vi "Configure Current Limit.vi"(8 "error in (no error)":errorcluster, 10 "Current Limit":dbl, 11 "Agilent 6xxx in":refnum<class "Agilent 6xxx.lvclass">) -> (0 "error out":errorcluster, 3 "Agilent 6xxx out":refnum<class "Agilent 6xxx.lvclass">)   [LabVIEW 2020, in "Agilent 6xxx.lvclass"]
uses:
  Agilent 6xxx.lvclass
  C:/Sandbox/RF Bench/Source Code/WiSpry Test Framework/Instruments/Instrument.lvclass
  C:/Sandbox/RF Bench/Source Code/WiSpry Test Framework/Instruments/Power Supply/Power Supply.lvclass
  Power Supply.lvclass/Power Supply.ctl
  Instrument.lvclass/Instrument.ctl
  Power Supply.lvclass
  Instrument.lvclass
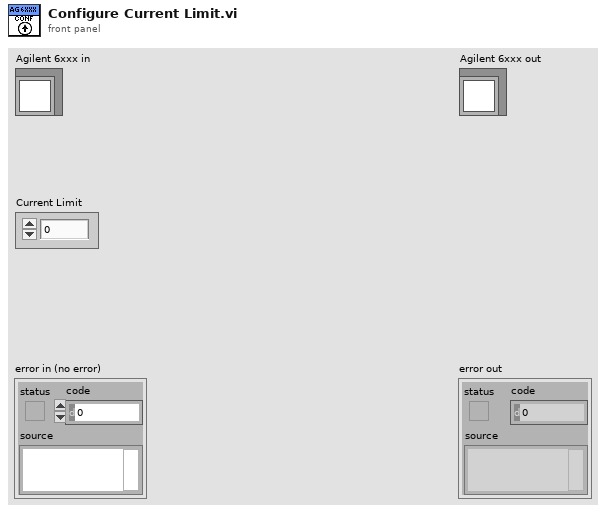
[diagram p1: front panel]
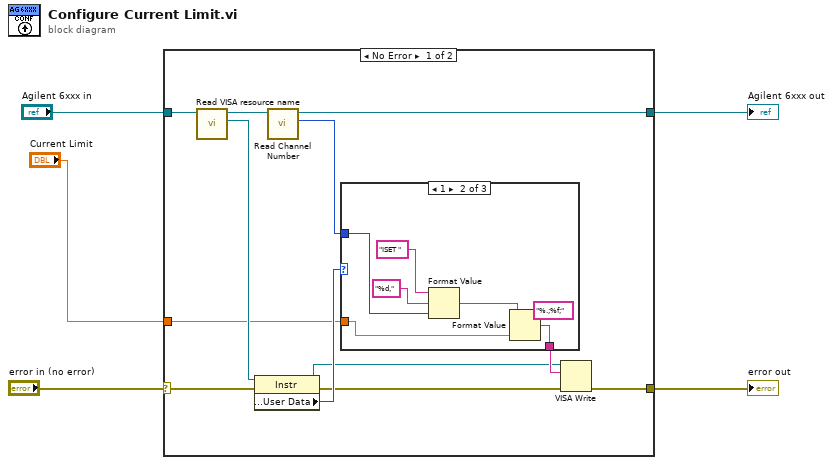
[diagram p0: block diagram]
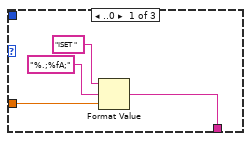
[diagram p2: hidden frame]
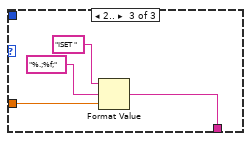
[diagram p3: hidden frame]
diagram:
  n1 = case shown="No Error" "error in (no error)" {
    selector: "error in (no error)" -> [w10 w33]
    tunnel: [w15 w34] -> w3
    tunnel: "Agilent 6xxx in" -> [w16 w34]
    tunnel: [w8 w33] -> w4
    tunnel: "Current Limit" -> [w6 _]
    frame No Error {
      n2 = call "Read VISA resource name.vi"("Instrument in"=w16) -> ("VISA resource name"=w9:refnum<visa-resource-name>, "Instrument out"=w17:refnum<class "Agilent 6xxx.lvclass">)  [unwired: 9 in]
      n3 = property class="Instr"(reference=w9, error in=w10) -> (reference out=w12:refnum<visa-resource-name>, error out=w11:errorcluster, "General Settings:User Data"=w13:u32)
      n4 = call "Read Channel Number.vi"("Power Supply in"=w17) -> ("Channel Number"=w7:u8, "Power Supply out"=w15:refnum<class "Agilent 6xxx.lvclass">)  [unwired: 9 in]
      n5 = case shown="1" w13 {
        tunnel: [w19 w27 w30] -> w14
        tunnel: w6 -> [w20 w24 w31]
        tunnel: w7 -> [_ w23 _]
        frame ..0 {
          n6 = Format Value(string ("")="ISET ", format string="%.;%fA;", value (0)=w20) -> (output string=w19:string)
        }
        frame 1 {
          n7 = Format Value(string ("")="ISET ", format string="%d,", value (0)=w23) -> (output string=w25:string)
          n8 = Format Value(string ("")=w25, format string="%.;%f;", value (0)=w24) -> (output string=w27:string)
        }
        frame 2.. {
          n9 = Format Value(string ("")="ISET ", format string="%.;%f;", value (0)=w31) -> (output string=w30:string)
        }
      }
      n10 = VISA Write(VISA resource name=w12, write buffer=w14, error in (no error)=w11) -> (error out=w8:errorcluster)  [unwired: 2 out]
    }
    frame Error {
    }
  }
  "error out" <- w4
  "Agilent 6xxx out" <- w3
